vi "Create PDFReader.vi"(0 "PDF Report IN":refnum<class "PDF Report Class.lvclass">, 2 "Action":T1, 5 "PdfReader IN":refnum<k24>, 7 "File and pages":T2={"Path"=path "", "Pages"="all", "Password"=""}, 11 "error in (no error)":errorcluster) -> (4 "PDF Report duplicate":refnum<class "PDF Report Class.lvclass">, 6 "PdfReader OUT":refnum<k24>, 8 "NumberOfPages":i32, 15 "error out":errorcluster)   [LabVIEW 2020, in "Exaprom PDF.lvlib"]
doc: "Version 1.1\nDeveloped by Jean-Marc Simard\nCopyright © 2012, Exaprom Inc.\nAll rights reserved.\nLicense: BSD\n\nWith iTextSharp 4.1.6 (http://itextsharp.sourceforge.net)\nunder Mozilla Public License Version 1.1\n(http://www.mozilla.org/MPL/MPL-1.1.html)"
uses:
  <userlib>/labview-PDF-writer-master/Exaprom PDF.lvlib
  <userlib>/labview-PDF-writer-master/LV Class/PDF Report Class/PDF Report Class.lvclass
  <userlib>/labview-PDF-writer-master/Controls/Concatenate Controls/PDF file to concatenate.ctl
  C:/Program Files (x86)/National Instruments/LabVIEW 2020/user.lib/labview-PDF-writer-master/DLL/itextsharp.dll
  DLL/itextsharp.dll
  <userlib>/labview-PDF-writer-master/Controls/General Controls/Create, open or close.ctl
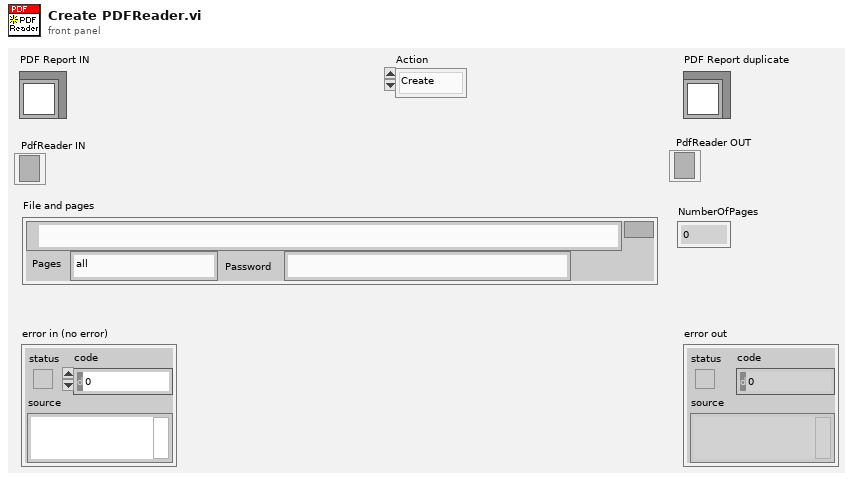
[diagram p1: front panel]
types:
  T1 = typedef "Exaprom PDF.lvlib/Create, open or close.ctl" = enum16{"Create", "Open", "Close"}
  T2 = typedef "Exaprom PDF.lvlib/PDF file to concatenate.ctl" = cluster{"Path":path, "Pages":string, "Password":string}
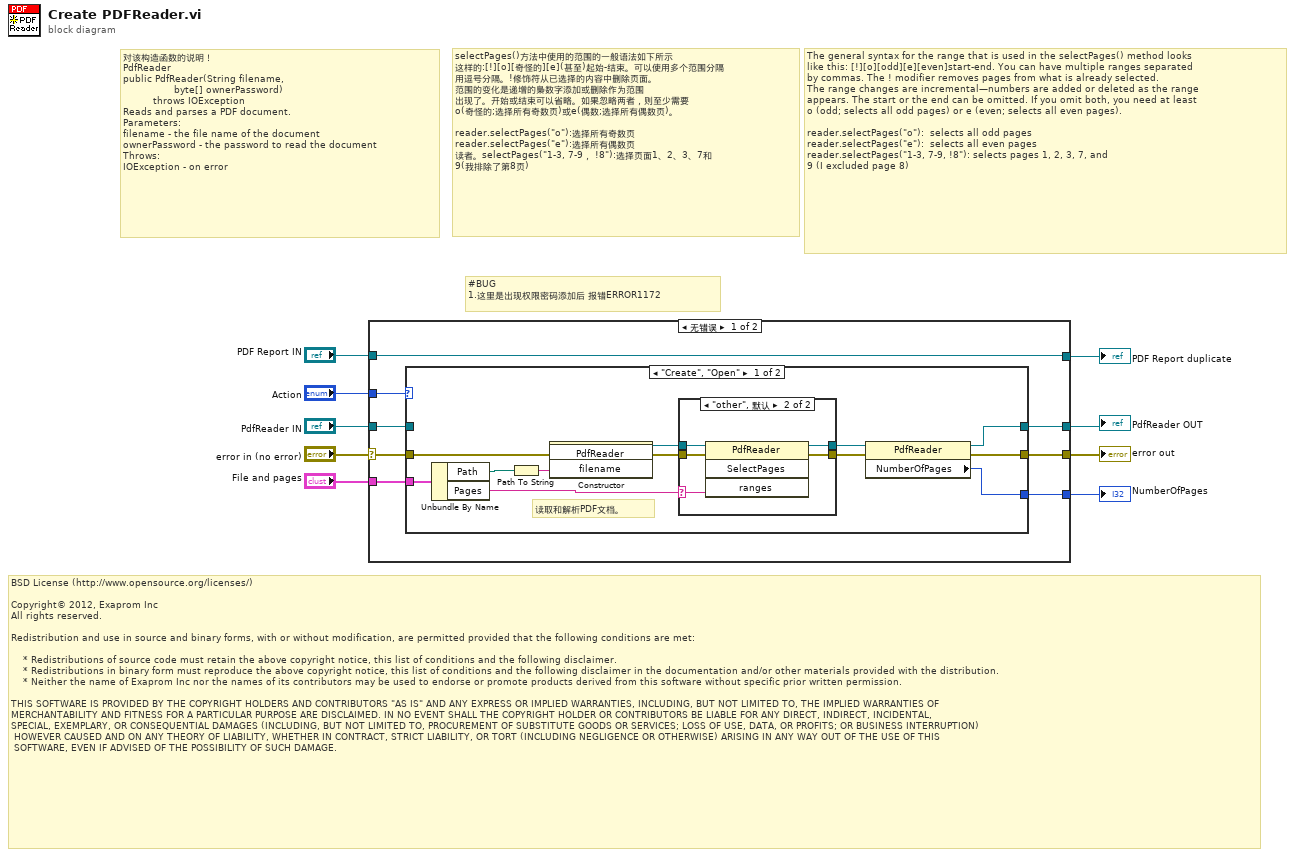
[diagram p0: block diagram]
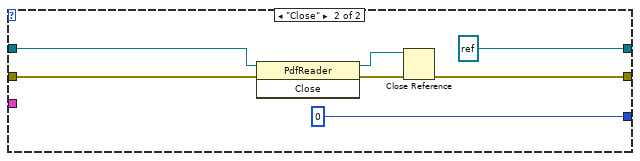
[diagram p3: hidden frame]
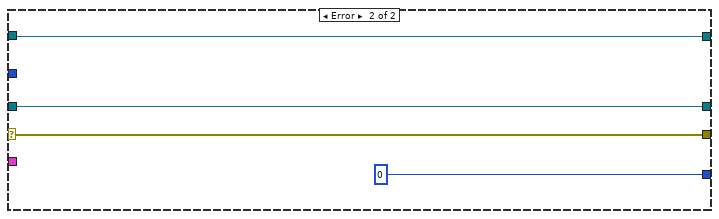
[diagram p4: hidden frame]
diagram:
  # "selectPages()方法中使用的范围的一般语法如下所示\n这样的:[!][o][奇怪的][e](甚至)起始-结束。可以使用多个范围分隔\n用逗号分隔。!修饰符从已选择的内容中删除页面。\n范围的变化是递增的梟数字添加或删除作为范围\n出现了。开始或结束可以省略。如果忽略两者，则至少需要\no(奇怪的;选择所有奇数页)或e(偶数;选择所有偶数页)。\n\nreader.selectPages(\"o\"):选择所有奇数页\nreader.selectPages(\"e\"):选择所有偶数页\n读者。selectPages(\"1-3, 7-9， !8\"):选择页面1、2、3、7和\n9(我排除了第8页)"
  # "对该构造函数的说明！\nPdfReader\npublic PdfReader(String filename,\n                 byte[] ownerPassword)\n          throws IOException\nReads and parses a PDF document.\nParameters:\nfilename - the file name of the document\nownerPassword - the password to read the document\nThrows:\nIOException - on error"
  # "#BUG  \n1.这里是出现权限密码添加后 报错ERROR1172"
  # "The general syntax for the range that is used in the selectPages() method looks\nlike this: [!][o][odd][e][even]start-end. You can have multiple ranges separated\nby commas. The ! modifier removes pages from what is already selected.\nThe range changes are incremental—numbers are added or deleted as the range\nappears. The start or the end can be omitted. If you omit both, you need at least\no (odd; selects all odd pages) or e (even; selects all even pages).\n\nreader.selectPages(\"o\"):  selects all odd pages\nreader.selectPages(\"e\"):  selects all even pages\nreader.selectPages(\"1-3, 7-9, !8\"): selects pages 1, 2, 3, 7, and\n9 (I excluded page 8)"
  # "BSD License (http://www.opensource.org/licenses/)\n\nCopyright© 2012, Exaprom Inc\nAll rights reserved.\n\nRedistribution and use in source and binary forms, with or without modification, are permitted provided that the following conditions are met:\n\n    * Redistributions of source code must retain the above copyright notice, this list of conditions and the following disclaimer.\n    * Redistributions in binary form must reproduce the above copyright notice, this list of conditions and the following disclaimer in the documentation and/or other materials provided with the distribution.\n    * Neither the name of Exaprom Inc nor the names of its contributors may be used to endorse or promote products derived from this software without specific prior written permission.\n\nTHIS SOFTWARE IS PROVIDED BY THE COPYRIGHT HOLDERS AND CONTRIBUTORS \"AS IS\" AND ANY EXPRESS OR IMPLIED WARRANTIES, INCLUDING, BUT NOT LIMITED TO, THE IMPLIED WARRANTIES OF \nMERCHANTABILITY AND FITNESS FOR A PARTICULAR PURPOSE ARE DISCLAIMED. IN NO EVENT SHALL THE COPYRIGHT HOLDER OR CONTRIBUTORS BE LIABLE FOR ANY DIRECT, INDIRECT, INCIDENTAL,\nSPECIAL, EXEMPLARY, OR CONSEQUENTIAL DAMAGES (INCLUDING, BUT NOT LIMITED TO, PROCUREMENT OF SUBSTITUTE GOODS OR SERVICES; LOSS OF USE, DATA, OR PROFITS; OR BUSINESS INTERRUPTION)\n HOWEVER CAUSED AND ON ANY THEORY OF LIABILITY, WHETHER IN CONTRACT, STRICT LIABILITY, OR TORT (INCLUDING NEGLIGENCE OR OTHERWISE) ARISING IN ANY WAY OUT OF THE USE OF THIS\n SOFTWARE, EVEN IF ADVISED OF THE POSSIBILITY OF SUCH DAMAGE."
  n1 = case shown="无错误" "error in (no error)" {
    selector: "error in (no error)" -> [w15 w47]
    tunnel: "PDF Report IN" -> [w17 w46]
    tunnel: [w17 w46] -> w8
    tunnel: [w14 w47] -> w7
    tunnel: "File and pages" -> [w16 _]
    tunnel: [w13 w45] -> w3
    tunnel: [w12 0 ("NumberOfPages")] -> w4
    tunnel: "Action" -> [w11 _]
    tunnel: "PdfReader IN" -> [w10 w45]
    frame No Error {
      n2 = case shown="\"Create\", \"Open\"" w11 {
        tunnel: w16 -> [w22 _]
        tunnel: w15 -> [w21 w43]
        tunnel: [w20 w39] -> w14
        tunnel: [w19 refnum<k24> refnum ("new reference")] -> w13
        tunnel: [w18 0 ("NumberOfPages")] -> w12
        tunnel: w10 -> [_ w41]
        frame "Create", "Open" {
          # "读取和解析PDF文档。"
          n3 = Unbundle By Name(w22) -> ("Path"=w28:path, "Pages"=w23:string)
          n4 = Path To String(path=w28) -> (string=w29:string)
          n5 = constructor class="PdfReader"(error in=w21, "filename"=w29) -> (reference out=w27:refnum<k24>, error out=w26:errorcluster)  [unwired: 2 in, 2 out]
          n6 = case shown="\"other\", 默认" w23 {
            selector: w23 -> [_ w32]
            tunnel: w27 -> [w31 w36]
            tunnel: w26 -> [w30 w35]
            tunnel: [w30 w34] -> w25
            tunnel: [w31 w33] -> w24
            frame "all" {
            }
            frame "other", Default {
              n7 = invoke class="PdfReader" method="SelectPages"(reference=w36, error in=w35, "ranges"=w32) -> (reference out=w33:refnum<k24>, error out=w34:errorcluster)  [unwired: 1 in, 2 out]
            }
          }
          n8 = property class="PdfReader"(reference=w24, error in=w25) -> (reference out=w19:refnum<k24>, error out=w20:errorcluster, "NumberOfPages"=w18:i32)
        }
        frame "Close" {
          n9 = invoke class="PdfReader" method="Close"(reference=w41, error in=w43) -> (reference out=w38:refnum<k24>, error out=w42:errorcluster)  [unwired: 1 in, 1 out]
          n10 = Close Reference(reference=w38, error in (no error)=w42) -> (error out=w39:errorcluster)
        }
      }
    }
    frame Error {
    }
  }
  "PDF Report duplicate" <- w8
  "error out" <- w7
  "NumberOfPages" <- w4
  "PdfReader OUT" <- w3
